vi "Interface-RS232.vi"() -> ()   [LabVIEW 2019]
uses:
  Documents/MEDAQLib-4.7.0.30086/Samples/LabView/MEDAQLib/MEDAQLib.lvlib
panel:
  in  "DLL-Path":path
  out "Last error text":string
  in  "COM Port":string="COM3"
  in  "Sensor type":string="ild1402"
  out "ScaledData":dbl[](graph)
  in  "stop":bool
  in  "Block size":i32=200
  # "1. Preparations\nPlease use Sensor tool to find sensor connected to your PC and get its interface/communication parameters."
  # "2. Inform MEDAQLib about sensor type and interface parameters.\nFor possible sensor type names see MEDAQLib.h or CreateSensorInstByName documentation in MEDAQLib.pdf\nCOM Port = Portname\nPlease note: this example expects to access the sensor with its default baudrate. You may need to insert another SetParameterInt VI to tell MEDAQLib about a changed baudrate."
  # "3. Start LabView execution"
  # "4.For stop please do not use LabView red stop button on toolbar, but the red STOP button below to be able to inform MEDAQLib about release of sensor instance information."
  # "Number of samples\nper transfered data block"
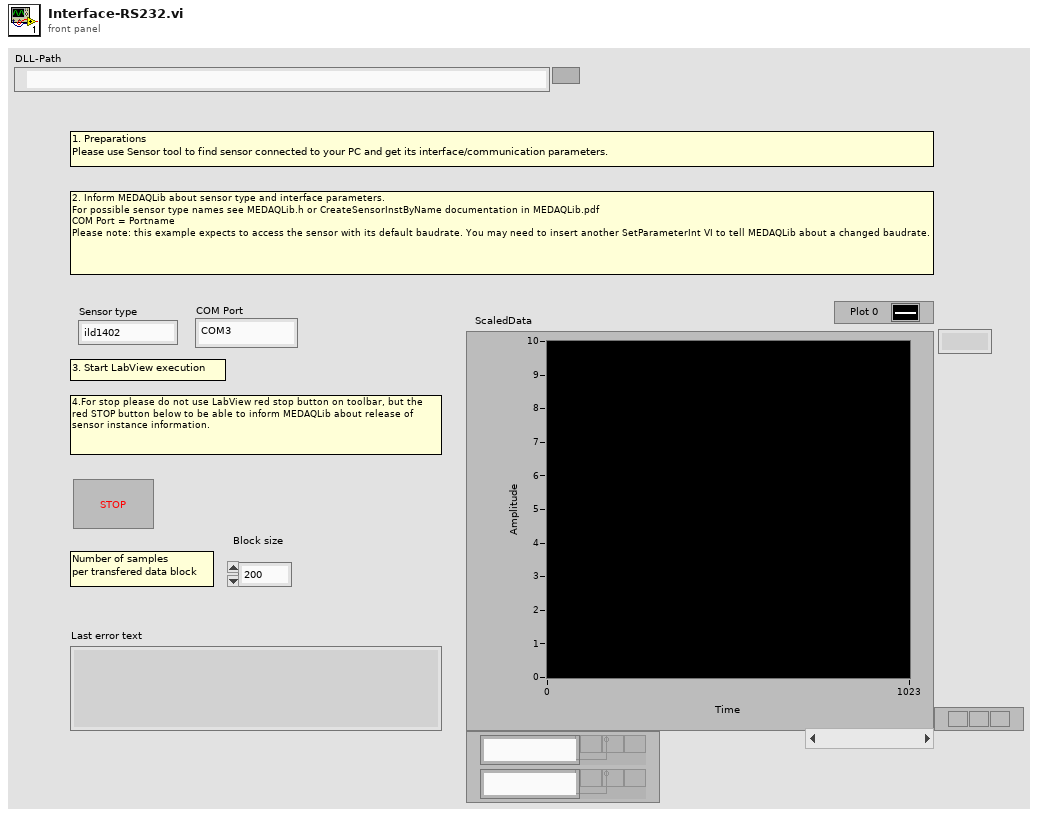
[diagram p1: front panel]
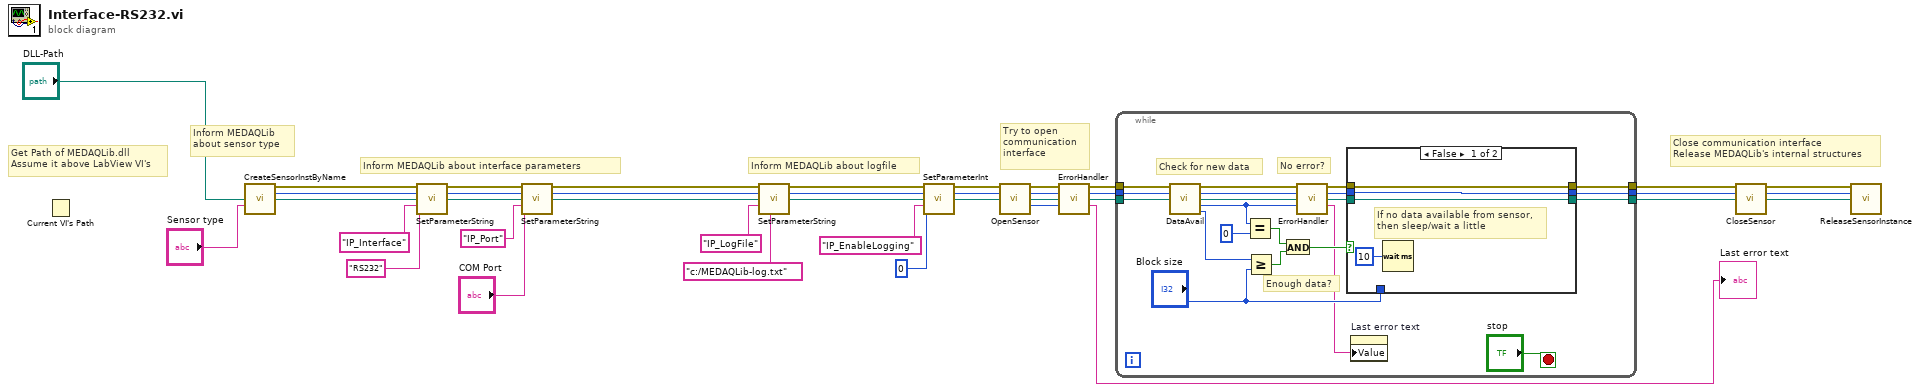
[diagram p0: block diagram]
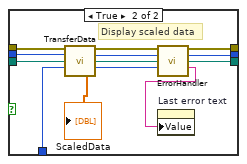
[diagram p2: hidden frame]
diagram:
  # "Close communication interface\nRelease MEDAQLib's internal structures"
  # "Try to open\ncommunication\ninterface"
  # "Inform MEDAQLib about logfile"
  # "Inform MEDAQLib about interface parameters"
  # "Inform MEDAQLib\nabout sensor type"
  # "Get Path of MEDAQLib.dll\nAssume it above LabView VI's"
  n1 = Current VI's Path() -> ()  [unwired: 1 out]
  n2 = call "CreateSensorInstByName.vi"("DLL-Path"="DLL-Path", "sensor"="Sensor type") -> ("Fehler (Ausgang)"=w38:errorcluster, "instanceHandle"=w37:u32, "DLL-Path"=w36:path)  [unwired: 1 in, 10 out]
  n3 = call "SetParameterString.vi"("Fehler (Eingang, kein Fehler)"=w38, "instanceHandle"=w37, "DLL-Path"=w36, "paramName"="IP_Interface", "paramValue"="RS232") -> ("Fehler (Ausgang)"=w33:errorcluster, "instanceHandle"=w32:u32, "DLL-Path"=w2:path)  [unwired: 8 out]
  n4 = call "SetParameterString.vi"("Fehler (Eingang, kein Fehler)"=w33, "instanceHandle"=w32, "DLL-Path"=w2, "paramName"="IP_Port", "paramValue"="COM Port") -> ("Fehler (Ausgang)"=w13:errorcluster, "instanceHandle"=w12:u32, "DLL-Path"=w11:path)  [unwired: 8 out]
  n5 = call "SetParameterString.vi"("Fehler (Eingang, kein Fehler)"=w13, "instanceHandle"=w12, "DLL-Path"=w11, "paramName"="IP_LogFile", "paramValue"="c:/MEDAQLib-log.txt") -> ("Fehler (Ausgang)"=w27:errorcluster, "instanceHandle"=w26:u32, "DLL-Path"=w25:path)  [unwired: 8 out]
  n6 = call "SetParameterInt.vi"("Fehler (Eingang, kein Fehler)"=w27, "instanceHandle"=w26, "DLL-Path"=w25, "paramName"="IP_EnableLogging", "paramValue"=0) -> ("Fehler (Ausgang)"=w22:errorcluster, "instanceHandle"=w21:u32, "DLL-Path"=w20:path)  [unwired: 8 out]
  n7 = call "OpenSensor.vi"("Fehler (Eingang, kein Fehler)"=w22, "instanceHandle"=w21, "DLL-Path"=w20) -> ("Fehler (Ausgang)"=w10:errorcluster, "instanceHandle"=w9:u32, "DLL-Path"=w8:path, "ERR_CODE"=w7:i32)  [unwired: 9 out]
  n8 = call "ErrorHandler.vi"("Fehler (Eingang, kein Fehler)"=w10, "instanceHandle"=w9, "DLL-Path"=w8, "ERR_CODE"=w7) -> ("Fehler (Ausgang)"=w6:errorcluster, "instanceHandle"=w5:u32, "DLL-Path"=w4:path, "errText"=→"Last error text":string)  [unwired: 8 out]
  n9 = while {
    tunnel: w6 -> [w60]
    tunnel: w5 -> [w59]
    tunnel: w4 -> [w58]
    tunnel: [w53] -> w19
    tunnel: [w52] -> w18
    tunnel: [w51] -> w17
    stop <- "stop" stop-if-true
    # "Enough data?"
    # "No error?"
    # "Check for new data"
    n10 = call "DataAvail.vi"("Fehler (Eingang, kein Fehler)"=w60, "instanceHandle"=w59, "DLL-Path"=w58) -> ("Fehler (Ausgang)"=w47:errorcluster, "instanceHandle"=w45:u32, "DLL-Path"=w43:path, "ERR_CODE"=w41:i32, "avail"=w57:i32)  [unwired: 8 out]
    n11 = Equal?(x=w41, y=0 ("x")) -> (x = y?=w54:bool)
    n12 = Greater Or Equal?(x=w57, y="Block size") -> (x >= y?=w50:bool)
    n13 = And(x=w54, y=w50) -> (x .and. y?=w55:bool)
    n14 = call "ErrorHandler.vi"("Fehler (Eingang, kein Fehler)"=w47, "instanceHandle"=w45, "DLL-Path"=w43, "ERR_CODE"=w41) -> ("Fehler (Ausgang)"=w46:errorcluster, "instanceHandle"=w44:u32, "DLL-Path"=w42:path, "errText"=w40:string)  [unwired: 8 out]
    n15 = case shown="False" w55 {
      tunnel: w46 -> [w64 w76]
      tunnel: w44 -> [w63 w77]
      tunnel: w42 -> [w62 w75]
      tunnel: [w64 w71] -> w53
      tunnel: [w63 w69] -> w52
      tunnel: [w62 w67] -> w51
      tunnel: "Block size" -> [_ w74]
      frame False {
        # "If no data available from sensor,\nthen sleep/wait a little"
        n16 = Wait (ms)(milliseconds to wait=u32 10 ("Zu wartende ms")) -> ()  [unwired: 1 out]
      }
      frame True {
        # "Display scaled data"
        n17 = call "TransferData.vi"("Fehler (Eingang, kein Fehler)"=w76, "instanceHandle"=w77, "DLL-Path"=w75, "maxValues"=w74) -> ("Fehler (Ausgang)"=w72:errorcluster, "instanceHandle"=w70:u32, "DLL-Path"=w68:path, "ERR_CODE"=w66:i32, "scaledData"=→"ScaledData":dbl[])  [unwired: 7 out]
        n18 = call "ErrorHandler.vi"("Fehler (Eingang, kein Fehler)"=w72, "instanceHandle"=w70, "DLL-Path"=w68, "ERR_CODE"=w66) -> ("Fehler (Ausgang)"=w71:errorcluster, "instanceHandle"=w69:u32, "DLL-Path"=w67:path, "errText"=w65:string)  [unwired: 8 out]
        n19 = property on="Last error text" class="Str"("Value"=w65) -> ()  [unwired: 2 in, 2 out]
      }
    }
    n20 = property on="Last error text" class="Str"("Value"=w40) -> ()  [unwired: 2 in, 2 out]
  }
  n21 = call "CloseSensor.vi"("Fehler (Eingang, kein Fehler)"=w19, "instanceHandle"=w18, "DLL-Path"=w17) -> ("Fehler (Ausgang)"=w16:errorcluster, "instanceHandle"=w15:u32, "DLL-Path"=w14:path)  [unwired: 10 out]
  n22 = call "ReleaseSensorInstance.vi"("Fehler (Eingang, kein Fehler)"=w16, "instanceHandle"=w15, "DLL-Path"=w14) -> ()  [unwired: 13 out]
